vi "play_testMatrix_load.vi"() -> ()   [LabVIEW 2014]
uses:
  <vilib>/rvi/interface/nirviMethod/nirviMethod.xnode
  <vilib>/rvi/errors/niLvFpgaMergeErrorWithErrorCode.vi
  <vilib>/rvi/interface/nirviReadWriteControl/nirviReadWriteControl.xnode
  <vilib>/Utility/error.llb/Error Cluster From Error Code.vi
  <vilib>/rvi/interface/Simulation/niFpgaSimulationCallBeginRW.vi
  <vilib>/rvi/errors/niLvFpgaAdjustHostInterfaceError.vi
  <vilib>/FPGAPlugInAG/Dynamic/niLvFpga_Reset_Dynamic.vi
  <vilib>/rvi/interface/nirviOpenFPGA/nirviOpenFPGA.xnode
  <vilib>/FPGAPlugInAG/Dynamic/niLvFpga_Run_Dynamic.vi
  <vilib>/rvi/interface/nirviCloseFPGA/nirviCloseFPGA.xnode
  FPGA Bitfiles/AFMsssinglematri_FPGATargetSPARTA_testMatrixloadDE_-SnzFq8Wpgc.lvbitx
  fpga_VIs/fpga_UnitTests/testMatrix_load_DELAY_fpga.vi
  <vilib>/FPGAPlugInAG/cRIO-9082/niLvFpga_Open_cRIO-9082.vi
  <vilib>/rvi/interface/common/dynamic/niFpgaDynamicAddResources.vi
  <vilib>/FPGAPlugInAG/Dynamic/niLvFpga_ConfigureFifo_Dynamic.vi
  NiFpgaLv.dll
  <vilib>/FPGAPlugInAG/Dynamic/niLvFpga_WriteFifo_Dynamic.vi
  <vilib>/FPGAPlugInAG/Dynamic/niLvFpga_Close_Dynamic.vi
panel:
  in  "Control Parameters path":path=path "C:/Users/arnold/Documents/MATLAB/AFM_SS/data/exp01Controls.csv"
  out "output array":dbl[](array[numeric])
  in  "Nd":i32
  out "Kdelay":sgl[](array[numeric])
  out "Ascol":sgl[](array[numeric])
  in  "Boolean":bool=TRUE
  out "Iter":i32
  out "B_out":sgl[](array[numeric])
  out "L_out":sgl[](array[numeric])
  out "K_out":sgl[](array[numeric])
  out "error constant":errorcluster
  out "Depth":i32
  out "Elements Remaing":i32
  out "All matrix 2":sgl[](array[numeric])
  in  "NS":i32
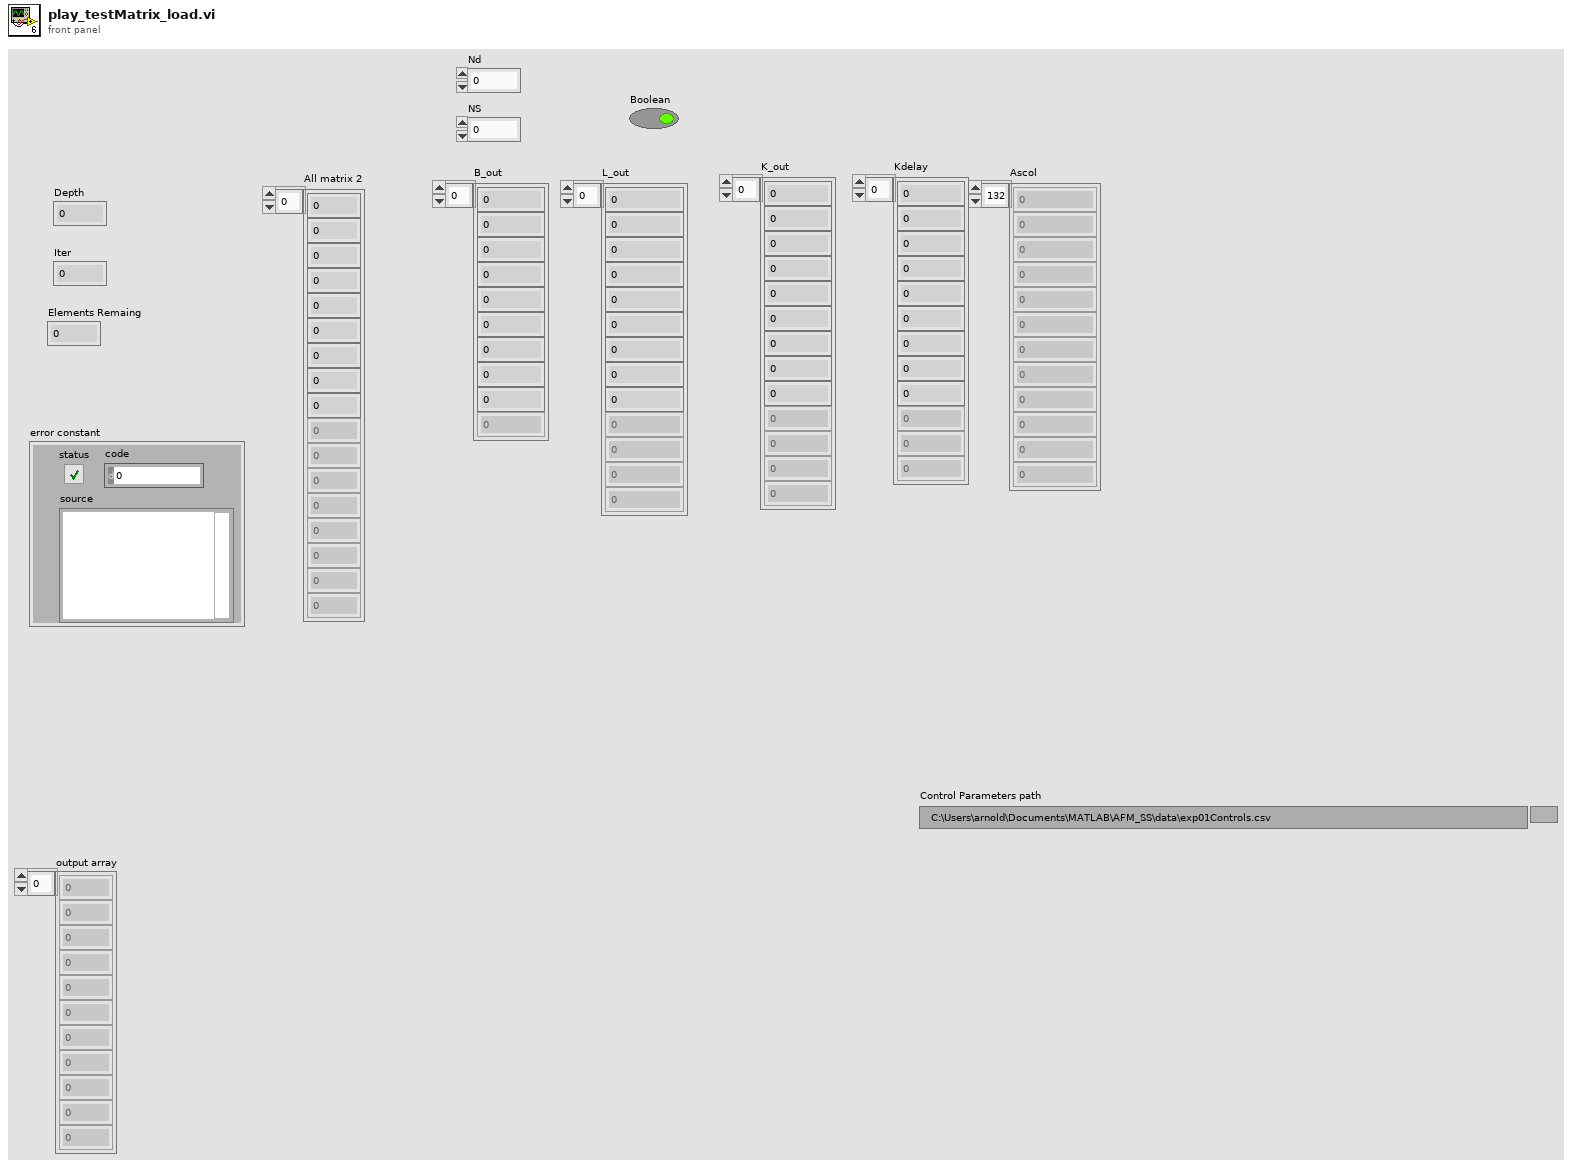
[diagram p1: front panel]
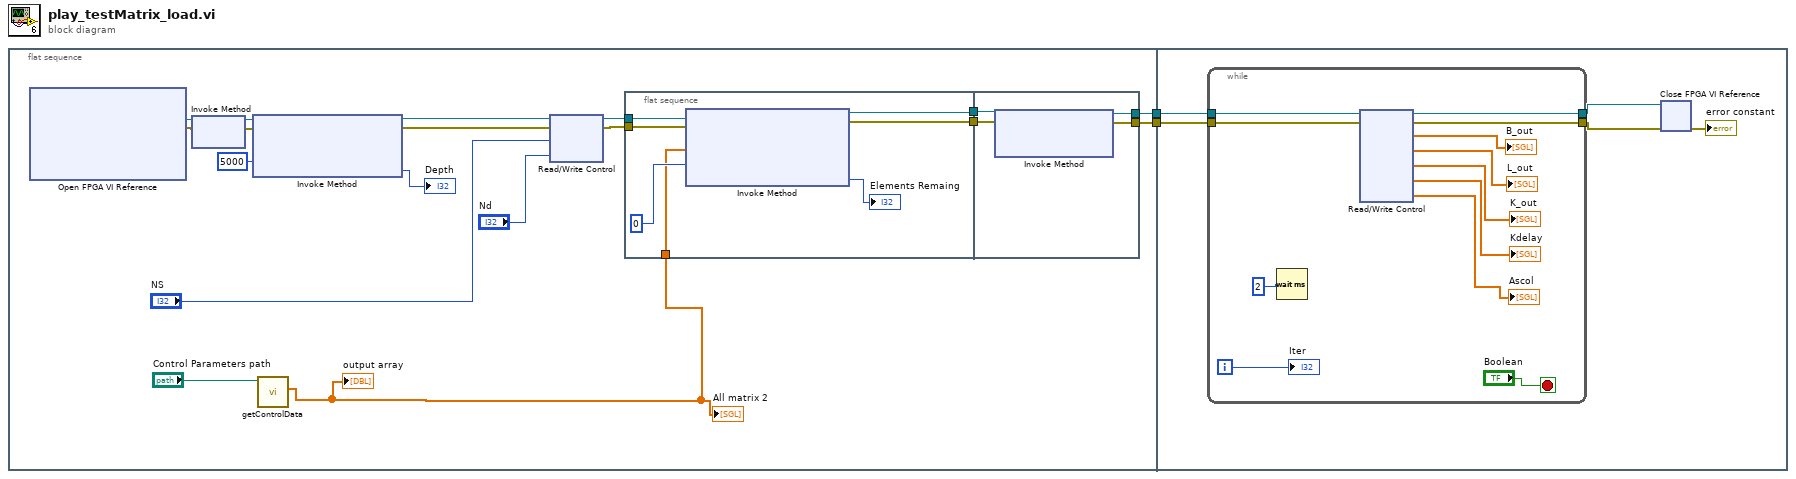
[diagram p0: block diagram]
diagram:
  n1 = flat-sequence {
    tunnel: [w12] -> w2
    tunnel: [w11] -> w1
    tunnel: w2 -> [w35]
    tunnel: w1 -> [w34]
    frame #0 {
      n2 = xnode "Open FPGA VI Reference"() -> ("FPGA VI Reference Out"=w16:refnum<k20>, "error out"=w17:errorcluster)  [unwired: 2 in]
      n3 = xnode "Invoke Method"("FPGA VI Reference In"=w16, "error in"=w17) -> ("FPGA VI Reference Out"=w19:refnum<k20>, "error out"=w20:errorcluster)
      n4 = xnode "Invoke Method"("FPGA VI Reference In"=w19, "error in"=w20, "Requested Depth"=5000) -> ("FPGA VI Reference Out"=w10:refnum<k20>, "error out"=w9:errorcluster, "Actual Depth"=→"Depth":u32)
      n5 = call "getControlData.vi"("system matricec path"="Control Parameters path") -> ("AllMatrix"=w3:dbl[])  [unwired: 9 in, 1 out]
      "All matrix 2" <- w3
      "output array" <- w3
      n6 = xnode "Read/Write Control"("FPGA VI Reference In"=w10, "error in"=w9, "NS"="NS", "ND"="Nd") -> ("FPGA VI Reference Out"=w14:refnum<k20>, "error out"=w13:errorcluster)
      n7 = flat-sequence {
        tunnel: w3 -> [w26]
        tunnel: w14 -> [w25]
        tunnel: w13 -> [w24]
        tunnel: [w23] -> w8
        tunnel: [w22] -> w7
        tunnel: w8 -> [w31]
        tunnel: w7 -> [w30]
        tunnel: [w29] -> w12
        tunnel: [w28] -> w11
        frame #0 {
          n8 = xnode "Invoke Method"("FPGA VI Reference In"=w25, "error in"=w24, "Data"=w26, "Timeout (ms)"=0) -> ("FPGA VI Reference Out"=w23:refnum<k20>, "error out"=w22:errorcluster, "Empty Elements Remaining"=→"Elements Remaing":u32)
        }
        frame #1 {
          n9 = xnode "Invoke Method"("FPGA VI Reference In"=w31, "error in"=w30) -> ("FPGA VI Reference Out"=w29:refnum<k20>, "error out"=w28:errorcluster)  [unwired: 1 in]
        }
      }
    }
    frame #1 {
      n10 = while {
        tunnel: [w43] -> w32
        tunnel: [w42] -> w33
        tunnel: w35 -> [w45]
        tunnel: w34 -> [w44]
        i -> [w48]
        stop <- "Boolean" stop-if-true
        n11 = Wait (ms)(milliseconds to wait=2) -> ()  [unwired: 1 out]
        n12 = xnode "Read/Write Control"("FPGA VI Reference In"=w45, "error in"=w44) -> ("FPGA VI Reference Out"=w43:refnum<k20>, "error out"=w42:errorcluster, "Bz"=→"B_out":sgl[], "L"=→"L_out":sgl[], "K"=→"K_out":sgl[], "Kdelay"=→"Kdelay":sgl[], "Aascol"=→"Ascol":sgl[])
        "Iter" <- w48
      }
      n13 = xnode "Close FPGA VI Reference"("FPGA VI Reference In"=w32, "error in"=w33) -> ("error out"=→"error constant":errorcluster)
    }
  }
